vi "PrepData.vi"(0 "object in":refnum<class "TDMSLogger_PowerScan.lvclass">, 1 "current time":timestamp, 2 "ChannelsWFIn":waveform(dbl)[](array[waveform]), 3 "AmplitudeAndVoltageSettings":T4, 4 "MeTecData":T3={"meTEC_CH2_Temperature Stability"=1, "meTEC_CH2_Act. Output Current [A]"=0.0, "meTEC_CH2_Act. Output Voltage [V]"=0.0, "meTEC_CH2_Object Temperature [°C]"=0.0, "meTEC_CH2_Sink Temperature [°C]"=0.0, "meTEC_CH1_Error Parameter"=0, "meTEC_CH1_Error Instance"=0, "meTEC_CH1_Error No."=0, "meTEC_CH1_Device Status"=1, "meTEC_CH1_Temperature Stability"=1, "meTEC_CH1_Act. Output Current [A]"=0.0, "meTEC_CH1_Act. Output Voltage [V]"=0.0, "meTEC_CH1_Object Temperature [°C]"=0.0, "meTEC_CH1_Sink Temperature [°C]"=0.0} {"meTEC_CH1_Sink Temperature [°C]" format="%.3f"; "meTEC_CH1_Object Temperature [°C]" format="%.3f"; "meTEC_CH1_Act. Output Voltage [V]" format="%.3f"; "meTEC_CH1_Act. Output Current [A]" format="%.3f"; "meTEC_CH1_Temperature Stability" items=["Temperature regulation is not active", "Is not stable", "Is stable"]; "meTEC_CH1_Device Status" items=["Initializing", "Ready", "Run", "Error", "Bootloader", "Reset in Progress"]; "meTEC_CH2_Sink Temperature [°C]" format="%.3f"; "meTEC_CH2_Object Temperature [°C]" format="%.3f"; "meTEC_CH2_Act. Output Voltage [V]" format="%.3f"; "meTEC_CH2_Act. Output Current [A]" format="%.3f"; "meTEC_CH2_Temperature Stability" items=["Temperature regulation is not active", "Is not stable", "Is stable"]}, 5 "error in (no error)":errorcluster, 7 "SetPower":dbl, 9 "MeasuredPower":dbl, 11 "AmplitudeOk":bool, 13 "WfgEnabled":cluster{"Ch1":bool, "Ch2":bool}) -> (14 "object out":refnum<class "TDMSLogger_PowerScan.lvclass">, 16 "Channel Names":string[](array[string]), 17 "Channels(WF)":waveform(dbl)[](array[waveform]), 19 "error out":errorcluster)   [LabVIEW 2023, in "TDMSLogger_PowerScan.lvclass"]
uses:
  TDMSLogger_PowerScan.lvclass
  TEC LabVIEW Control Software v0.14/Source/LV Source/[meerstetter engineering TE Cooling]/TypeDefs/meTEC_ID 1200_Temperature is Stable.ctl
  TEC LabVIEW Control Software v0.14/Source/LV Source/[meerstetter engineering TE Cooling]/TypeDefs/meTEC_ID 104_Device Status.ctl
  <vilib>/measure/matone.llb/Extract Single Tone Information 1 Chan.vi
  <vilib>/measure/NI_MAPro.lvlib
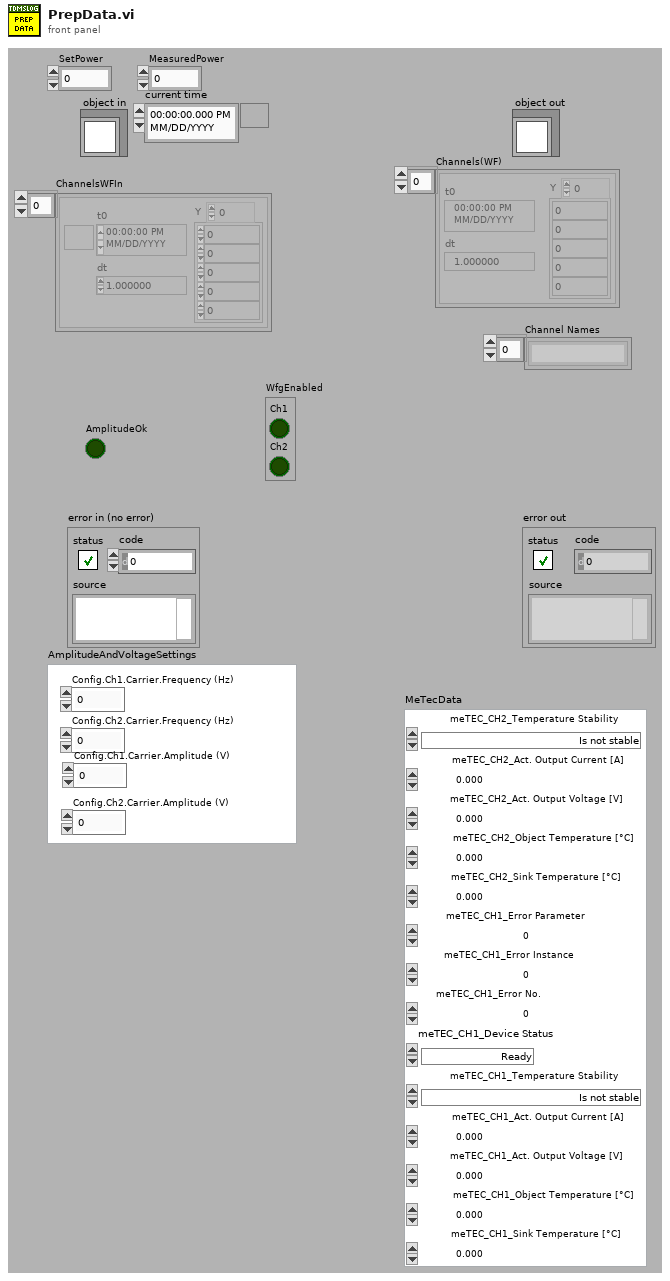
[diagram p1: front panel]
types:
  T1 = typedef "meTEC_ID 1200_Temperature is Stable.ctl" = i32
  T2 = typedef "meTEC_ID 104_Device Status.ctl" = i32
  T3 = cluster{"meTEC_CH2_Temperature Stability":T1, "meTEC_CH2_Act. Output Current [A]":dbl, "meTEC_CH2_Act. Output Voltage [V]":dbl, "meTEC_CH2_Object Temperature [°C]":dbl, "meTEC_CH2_Sink Temperature [°C]":dbl, "meTEC_CH1_Error Parameter":i32, "meTEC_CH1_Error Instance":i32, "meTEC_CH1_Error No.":i32, "meTEC_CH1_Device Status":T2, "meTEC_CH1_Temperature Stability":T1, "meTEC_CH1_Act. Output Current [A]":dbl, "meTEC_CH1_Act. Output Voltage [V]":dbl, "meTEC_CH1_Object Temperature [°C]":dbl, "meTEC_CH1_Sink Temperature [°C]":dbl}
  T4 = cluster{"Config.Ch1.Carrier.Frequency (Hz)":dbl, "Config.Ch2.Carrier.Frequency (Hz)":dbl, "Config.Ch1.Carrier.Amplitude (V)":dbl, "Config.Ch2.Carrier.Amplitude (V)":dbl}
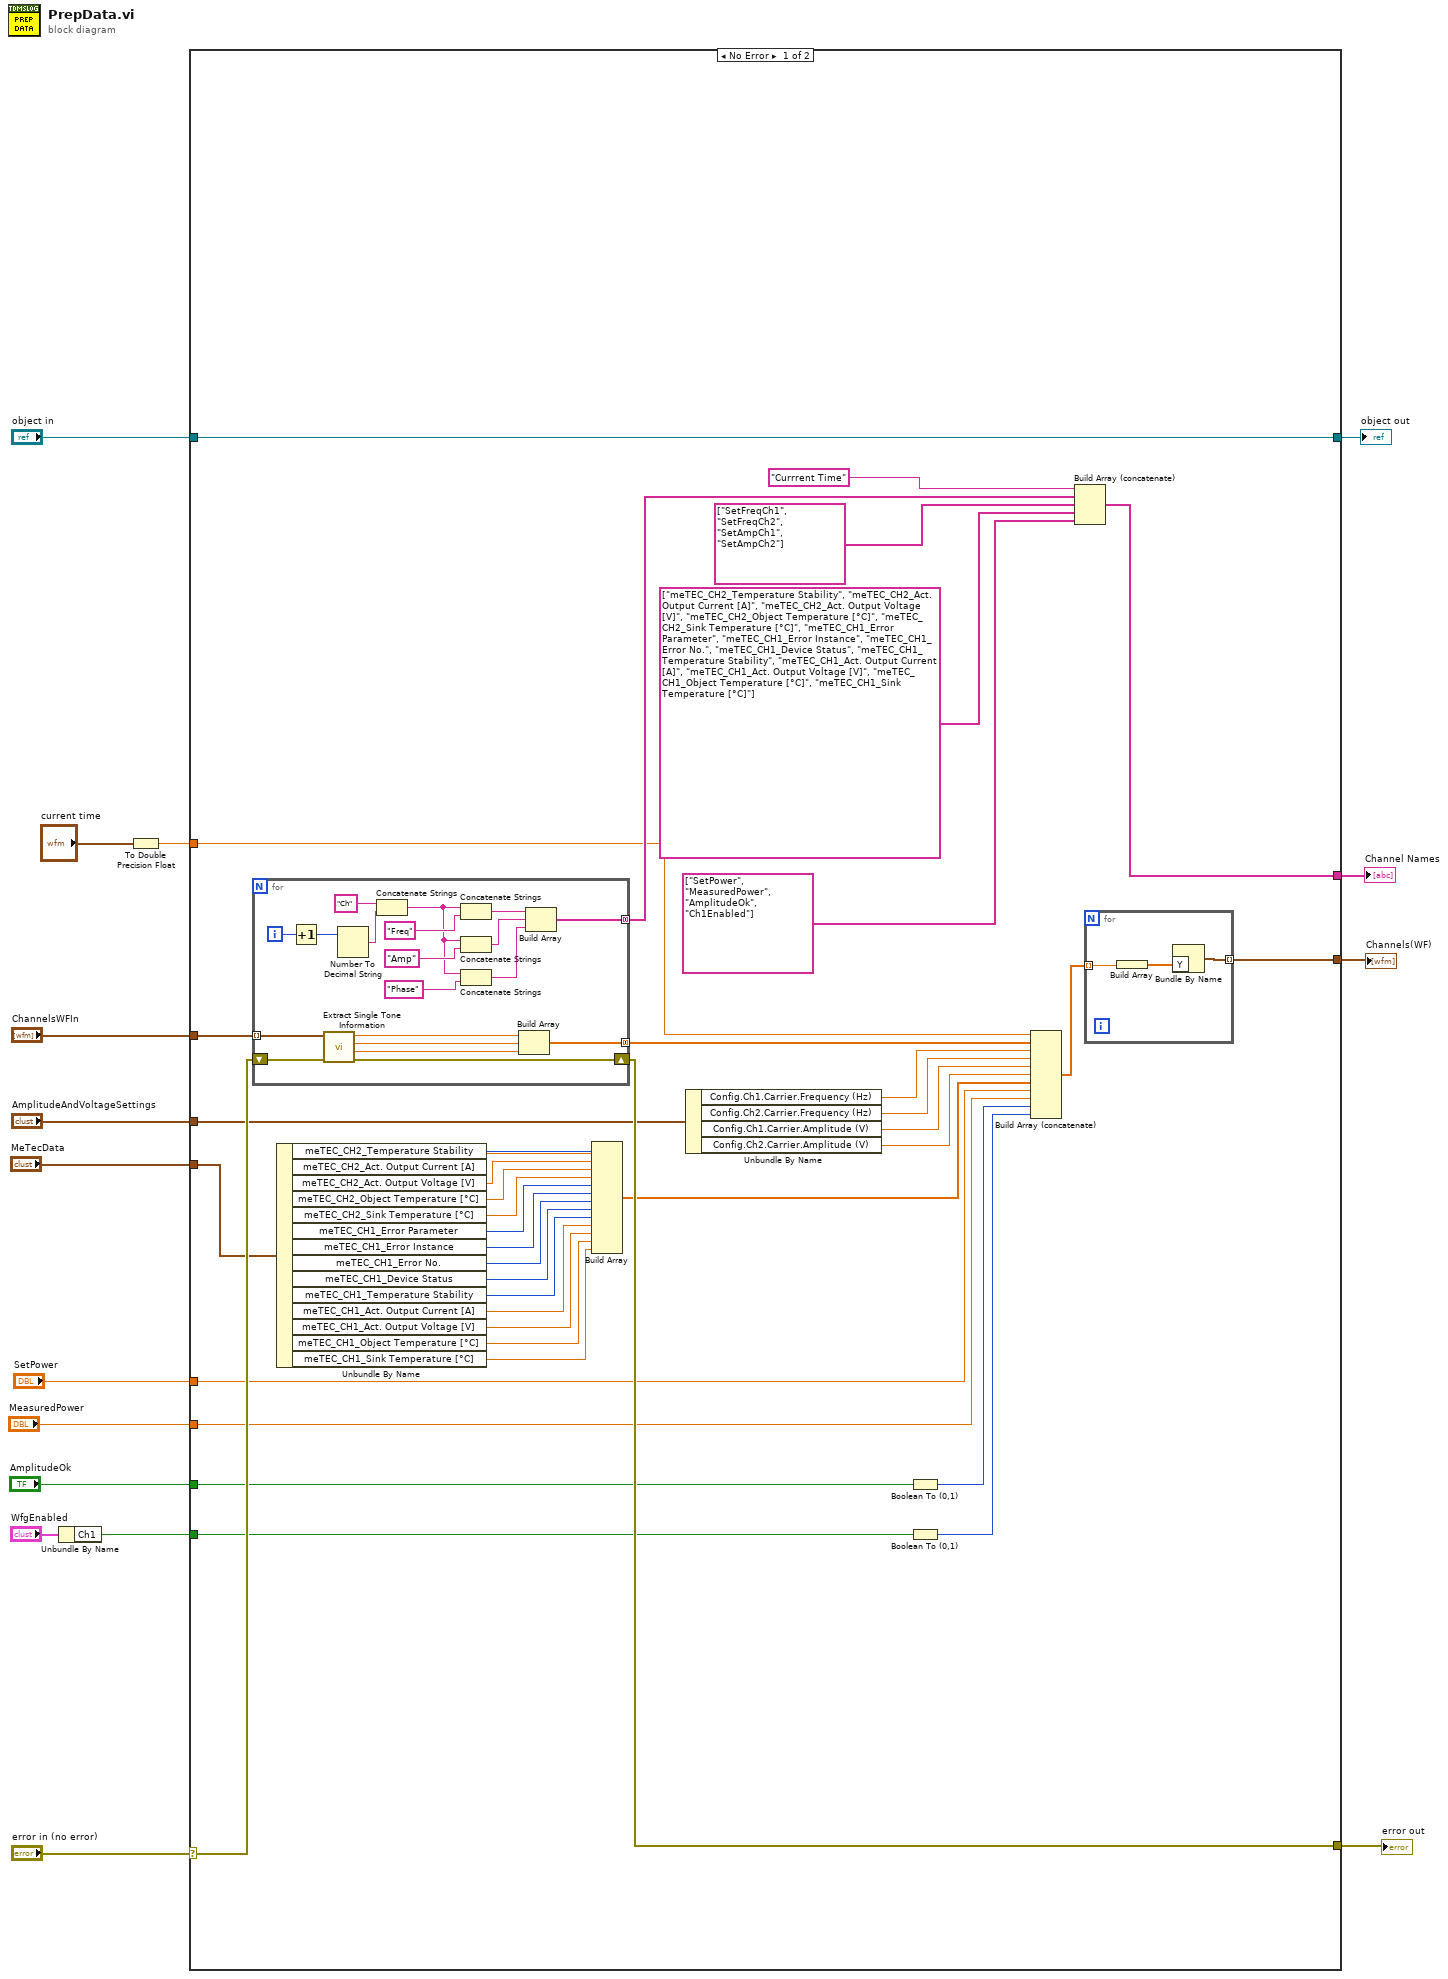
[diagram p0: block diagram]
diagram:
  n1 = Unbundle By Name("WfgEnabled") -> ("Ch1"=w3:bool)
  n2 = To Double Precision Float(number="current time") -> (double precision float=w2:dbl)
  n3 = case shown="No Error" "error in (no error)" {
    selector: "error in (no error)" -> [w47 w81]
    tunnel: [w46 w81] -> w15
    tunnel: [w57 w80] -> w13
    tunnel: "object in" -> [w57 w80]
    tunnel: [w55 _] -> w12
    tunnel: [w51 _] -> w11
    tunnel: "AmplitudeAndVoltageSettings" -> [w29 _]
    tunnel: "ChannelsWFIn" -> [w49 _]
    tunnel: "MeTecData" -> [w43 _]
    tunnel: w2 -> [w26 _]
    tunnel: "SetPower" -> [w23 _]
    tunnel: "MeasuredPower" -> [w22 _]
    tunnel: "AmplitudeOk" -> [w20 _]
    tunnel: w3 -> [w18 _]
    frame No Error {
      n4 = for {
        tunnel: [w71] -> w50 mode=concatenating
        shift-right: [w66] -> w46
        shift-left: w47 -> [w67]
        tunnel: [w62] -> w48 mode=concatenating
        tunnel: w49 -> [w61] mode=indexing
        i -> [w77]
        n5 = Increment(x=w77) -> (x+1=w72:i32)
        n6 = call-poly <vilib>:"Extract Single Tone Information.vi"("error in (no error)"=w67, "time signal in"=w61) -> ("error out"=w66:errorcluster, "detected phase (deg)"=w63:dbl, "detected amplitude"=w64:dbl, "detected frequency"=w65:dbl)  [unwired: 4 in, 2 out]
        n7 = Number To Decimal String(number=w72) -> (decimal integer string=w78:string)  [unwired: 1 in]
        n8 = Concatenate Strings("Ch" ("string"), w78) -> (w70:string)
        n9 = Concatenate Strings(w70, "Freq") -> (w74:string)
        n10 = Concatenate Strings(w70, "Amp") -> (w73:string)
        n11 = Concatenate Strings(w70, "Phase") -> (w68:string)
        n12 = Build Array(w65, w64, w63) -> (w62:dbl[])
        n13 = Build Array(w74, w73, w68) -> (w71:string[])
      }
      n14 = Unbundle By Name(w43) -> ("meTEC_CH2_Temperature Stability"=w42:T1, "meTEC_CH2_Act. Output Current [A]"=w41:dbl, "meTEC_CH2_Act. Output Voltage [V]"=w40:dbl, "meTEC_CH2_Object Temperature [°C]"=w39:dbl, "meTEC_CH2_Sink Temperature [°C]"=w38:dbl, "meTEC_CH1_Error Parameter"=w37:i32, "meTEC_CH1_Error Instance"=w36:i32, "meTEC_CH1_Error No."=w35:i32, "meTEC_CH1_Device Status"=w34:T2, "meTEC_CH1_Temperature Stability"=w33:T1, "meTEC_CH1_Act. Output Current [A]"=w32:dbl, "meTEC_CH1_Act. Output Voltage [V]"=w31:dbl, "meTEC_CH1_Object Temperature [°C]"=w30:dbl, "meTEC_CH1_Sink Temperature [°C]"=w21:dbl)
      n15 = Build Array(w42, w41, w40, w39, w38, w37, w36, w35, w34, w33, w32, w31, w30, w21) -> (w28:dbl[])
      n16 = Unbundle By Name(w29) -> ("Config.Ch1.Carrier.Frequency (Hz)"=w54:dbl, "Config.Ch2.Carrier.Frequency (Hz)"=w53:dbl, "Config.Ch1.Carrier.Amplitude (V)"=w45:dbl, "Config.Ch2.Carrier.Amplitude (V)"=w44:dbl)
      n17 = Boolean To (0,1)(Boolean=w20) -> (0, 1=w19:i16)
      n18 = Boolean To (0,1)(Boolean=w18) -> (0, 1=w17:i16)
      n19 = Build Array (concatenate)(w26, w48, w54, w53, w45, w44, w28, w23, w22, w19, w17) -> (w56:dbl[])
      n20 = Build Array (concatenate)("Currrent Time", w50, string[] ["SetFreqCh1", "SetFreqCh2", "SetAmpCh1", "SetAmpCh2"] ("channel name(s) in (Untitled)"), string[] ["meTEC_CH2_Temperature Stability", "meTEC_CH2_Act. Output Current [A]", "meTEC_CH2_Act. Output Voltage [V]", "meTEC_CH2_Object Temperature [°C]", "meTEC_CH2_Sink Temperature [°C]", "meTEC_CH1_Error Parameter", "meTEC_CH1_Error Instance", "meTEC_CH1_Error No.", "meTEC_CH1_Device Status", "meTEC_CH1_Temperature Stability", "meTEC_CH1_Act. Output Current [A]", "meTEC_CH1_Act. Output Voltage [V]", "meTEC_CH1_Object Temperature [°C]", "meTEC_CH1_Sink Temperature [°C]"] ("Array"), string[] ["SetPower", "MeasuredPower", "AmplitudeOk", "Ch1Enabled"] ("channel name(s) in (Untitled)")) -> (w51:string[])
      n21 = for {
        tunnel: w56 -> [w60] mode=indexing
        tunnel: [w58] -> w55 mode=indexing
        n22 = Build Array(w60) -> (w59:dbl[])
        n23 = Bundle By Name("Y"=w59) -> (w58:waveform(dbl))  [unwired: 1 in]
      }
    }
    frame Error {
    }
  }
  "error out" <- w15
  "object out" <- w13
  "Channels(WF)" <- w12
  "Channel Names" <- w11
